vi "execute.vi"(10 "task token":refnum<class "null task token.lvclass">, 11 "wait action in":refnum<class "wait action.lvclass">) -> (3 "result":refnum<class "result.lvclass">)   [LabVIEW 2013, in "wait action.lvclass"]
uses:
  wait action.lvclass
  result/result.lvclass
  task token/null task token.lvclass
  action/action.lvclass/action.ctl
  action/action.lvclass
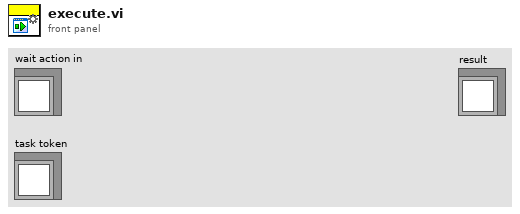
[diagram p1: front panel]
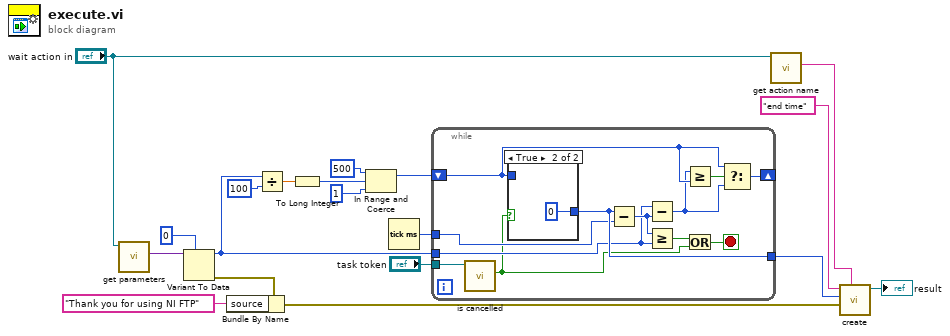
[diagram p0: block diagram]
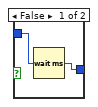
[diagram p2: hidden frame]
diagram:
  n1 = call "get parameters.vi"("action in"="wait action in") -> ("parameters"=w19:variant)  [unwired: 9 in, 1 out]
  n2 = Variant To Data(type=u32 0 ("milliseconds to wait"), Variant=w19) -> (data=w1:u32, error out=w15:errorcluster)  [unwired: 1 in]
  n3 = Bundle By Name(cluster=w15, "source"="Thank you for using NI FTP") -> (w12:errorcluster)
  n4 = Divide(x=w1, y=u32 100) -> (x/y=w6:dbl)
  n5 = To Long Integer(number=w6) -> (32bit integer=w5:i32)
  n6 = In Range and Coerce(upper limit=500, x=w5, lower limit=1) -> (coerced(x)=w2:i32)  [unwired: 1 out]
  n7 = Tick Count (ms)() -> (millisecond timer value=w8:u32)
  n8 = while {
    tunnel: [w30] -> w11
    tunnel: "task token" -> [w31]
    tunnel: w8 -> [w29]
    tunnel: w1 -> [w25]
    shift-right: [w22] -> _
    shift-left: w2 -> [w23]
    stop <- w28 stop-if-true
    n9 = call-dynamic "is cancelled.vi"("null task token in"=w31) -> ("cancelled?"=w20:bool)  [unwired: 9 in, 1 out]
    n10 = case shown="True" w20 {
      tunnel: [w33 u32 0 ("millisecond timer value")] -> w30
      tunnel: w23 -> [w32 _]
      frame False {
        n11 = Wait (ms)(milliseconds to wait=w32) -> (millisecond timer value=w33:u32)
      }
      frame True {
      }
    }
    n12 = Subtract(x=w30, y=w29) -> (x-y=w26:u32)
    n13 = Subtract(x=w25, y=w26) -> (x-y=w21:u32)
    n14 = Greater Or Equal?(x=w26, y=w25) -> (x >= y?=w27:bool)
    n15 = Greater Or Equal?(x=w21, y=w23) -> (x >= y?=w24:bool)
    n16 = Or(x=w27, y=w20) -> (x .or. y?=w28:bool)
    n17 = Select(t=w23, s=w24, f=w21) -> (s? t:f=w22:u32)
  }
  n18 = call "get action name.vi"("action in"="wait action in") -> ("action name"=w13:string)  [unwired: 9 in, 1 out]
  n19 = call "create.vi"("generating action"=w13, "error"=w12, "data"=w11, "data ID"="end time") -> ("result out"=→"result":refnum<class "result.lvclass">)  [unwired: 7 in]
